vi "SwerveDefensiveCalculations.vi"(9 "J2X":dbl, 11 "Pivot Module":i32) -> (0 "Magnitude 3":dbl, 1 "Magnitude 2":dbl, 2 "Magnitude 1":dbl, 3 "Magnitude 0":dbl, 4 "Wheel Angle 3":dbl, 5 "Wheel Angle 1":dbl, 6 "Wheel Angle 2":dbl, 7 "Wheel Angle 0":dbl)   [LabVIEW 2019]
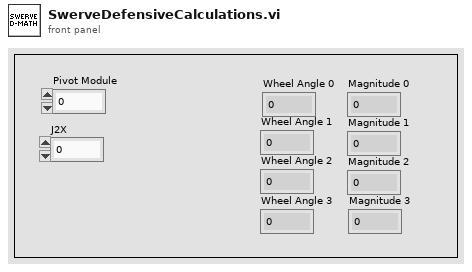
[diagram p1: front panel]
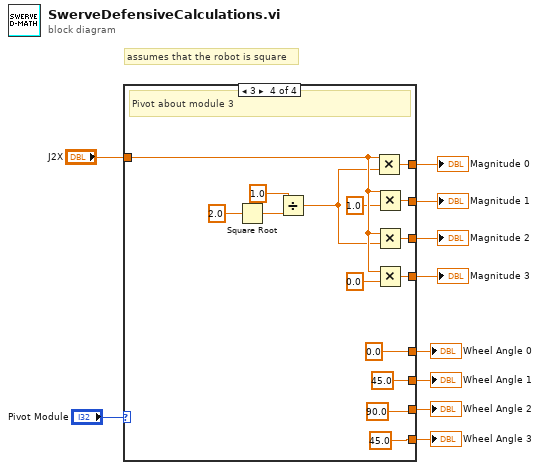
[diagram p0: block diagram]
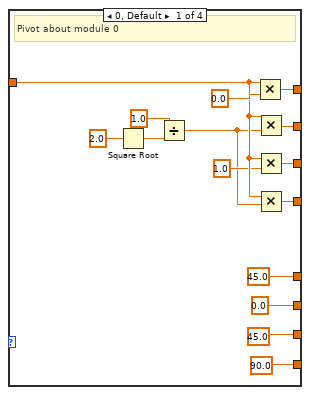
[diagram p2: hidden frame]
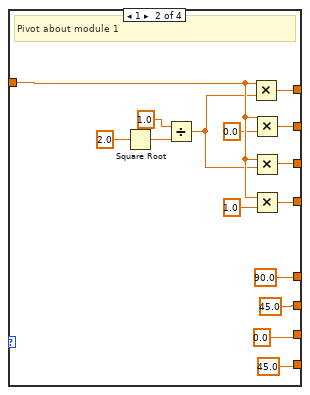
[diagram p3: hidden frame]
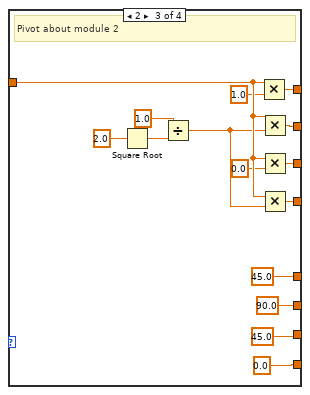
[diagram p4: hidden frame]
diagram:
  # "assumes that the robot is square"
  n1 = case shown="3" "Pivot Module" {
    tunnel: [45.0 90.0 45.0 0.0] -> w9
    tunnel: [0.0 45.0 90.0 45.0] -> w8
    tunnel: [45.0 0.0 45.0 90.0] -> w7
    tunnel: [90.0 45.0 0.0 45.0] -> w6
    tunnel: "J2X" -> [w20 w37 w52 w67]
    tunnel: [w25 w32 w47 w66] -> w5
    tunnel: [w23 w31 w46 w65] -> w4
    tunnel: [w22 w30 w45 w64] -> w3
    tunnel: [w21 w29 w44 w63] -> w2
    frame 0, Default {
      # "Pivot about module 0"
      n2 = Square Root(x=2.0) -> (sqrt(x)=w17:dbl)
      n3 = Divide(x=1.0, y=w17) -> (x/y=w15:dbl)
      n4 = Multiply(x=w20, y=0.0) -> (x*y=w25:dbl)
      n5 = Multiply(x=w20, y=w15) -> (x*y=w23:dbl)
      n6 = Multiply(x=w20, y=1.0) -> (x*y=w22:dbl)
      n7 = Multiply(x=w20, y=w15) -> (x*y=w21:dbl)
    }
    frame 1 {
      # "Pivot about module 1"
      n8 = Square Root(x=2.0) -> (sqrt(x)=w40:dbl)
      n9 = Divide(x=1.0, y=w40) -> (x/y=w26:dbl)
      n10 = Multiply(x=w37, y=w26) -> (x*y=w32:dbl)
      n11 = Multiply(x=w37, y=0.0) -> (x*y=w31:dbl)
      n12 = Multiply(x=w37, y=w26) -> (x*y=w30:dbl)
      n13 = Multiply(x=w37, y=1.0) -> (x*y=w29:dbl)
    }
    frame 2 {
      # "Pivot about module 2"
      n14 = Square Root(x=2.0) -> (sqrt(x)=w54:dbl)
      n15 = Divide(x=1.0, y=w54) -> (x/y=w41:dbl)
      n16 = Multiply(x=w52, y=1.0) -> (x*y=w47:dbl)
      n17 = Multiply(x=w52, y=w41) -> (x*y=w46:dbl)
      n18 = Multiply(x=w52, y=0.0) -> (x*y=w45:dbl)
      n19 = Multiply(x=w52, y=w41) -> (x*y=w44:dbl)
    }
    frame 3 {
      # "Pivot about module 3"
      n20 = Square Root(x=2.0) -> (sqrt(x)=w69:dbl)
      n21 = Divide(x=1.0, y=w69) -> (x/y=w56:dbl)
      n22 = Multiply(x=w67, y=w56) -> (x*y=w66:dbl)
      n23 = Multiply(x=w67, y=1.0) -> (x*y=w65:dbl)
      n24 = Multiply(x=w67, y=w56) -> (x*y=w64:dbl)
      n25 = Multiply(x=w67, y=0.0) -> (x*y=w63:dbl)
    }
  }
  "Wheel Angle 0" <- w9
  "Wheel Angle 1" <- w8
  "Wheel Angle 2" <- w7
  "Wheel Angle 3" <- w6
  "Magnitude 0" <- w5
  "Magnitude 1" <- w4
  "Magnitude 2" <- w3
  "Magnitude 3" <- w2
